vi "sub_simulation_main.vi"(8 "error in":errorcluster) -> (0 "error out":errorcluster)   [LabVIEW 2016]
uses:
  ctl/UI_cmd-ctl.ctl
  ctl/q_data.ctl
  Global.vi
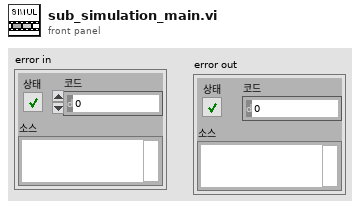
[diagram p1: front panel]
types:
  T1 = typedef "UI_cmd-ctl.ctl" = enum16{"default", "create", "read"}
  T2 = typedef "q_data.ctl" = cluster{"Strain raw wf":waveform(dbl)[], "vacuum raw wf":waveform(dbl), "IR raw 2d":i16[][]}
  T3 = cluster{"simulation file path":path, "simulation speed":u32}
  T4 = typedef "UI_ctl2.ctl" = cluster{"simulation status":refnum<vi>}
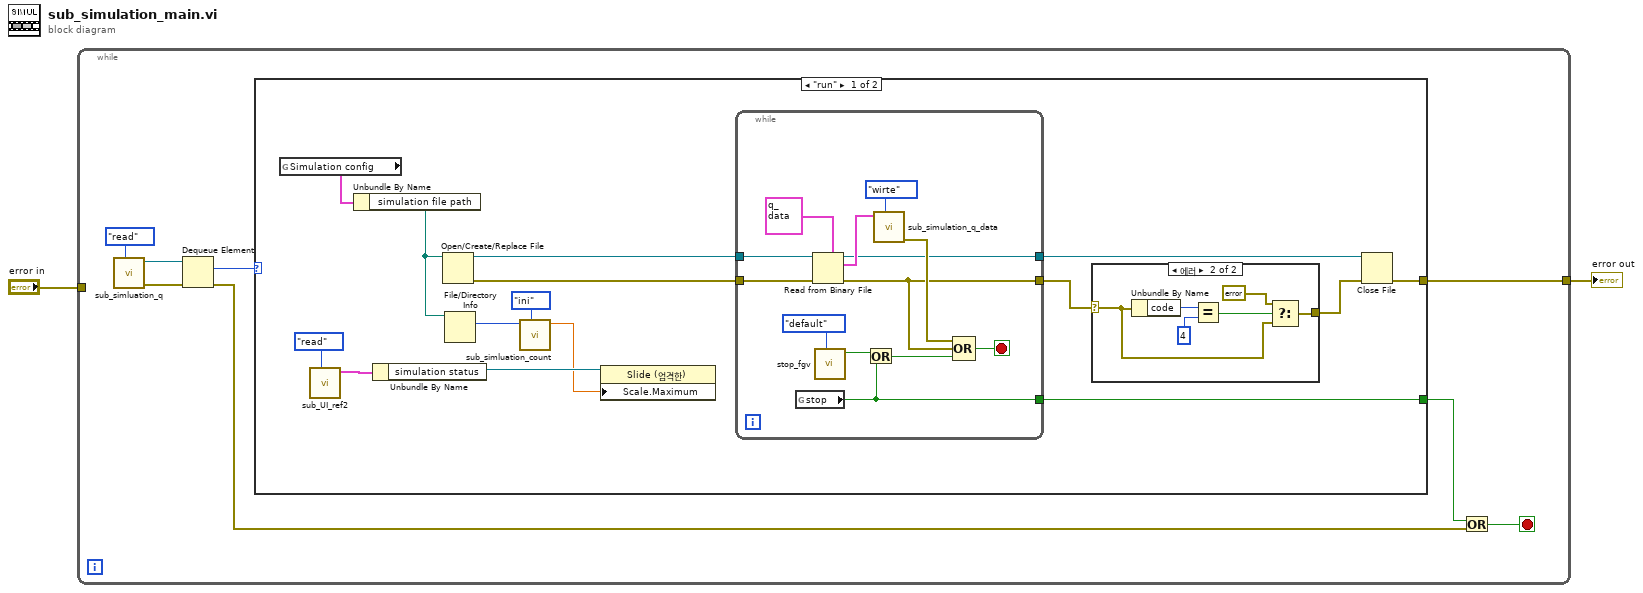
[diagram p0: block diagram]
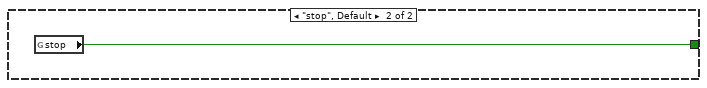
[diagram p3: hidden frame]
diagram:
  n1 = while {
    tunnel: "error in" -> [_]
    tunnel: [w3] -> w1
    stop <- w4 stop-if-true
    n2 = call "sub_simluation_q.vi"("cmd"=enum16{"create", "write", "read", "close"}."read") -> ("error out"=w9:errorcluster, "queue out"=w8:refnum<queue>)  [unwired: 9 in]
    n3 = Dequeue Element(queue=w8, error in (no error)=w9) -> (element=w7:enum16{"run", "stop"}, error out=w5:errorcluster)  [unwired: 1 in, 2 out]
    n4 = case shown="\"run\"" w7 {
      tunnel: [w22 w46] -> w6
      tunnel: [w21 _] -> w3
      frame "run" {
        n5 = global read "Global.vi" "Simulation config"() -> (w18:T3)
        n6 = call "sub_UI_ref2.vi"("cmd"=UI_cmd-ctl."read") -> ("UI ctl2 out"=w15:T4)  [unwired: 10 in]
        n7 = Unbundle By Name(w18) -> ("simulation file path"=w17:path)
        n8 = Unbundle By Name(w15) -> ("simulation status"=w14:refnum<vi>)
        n9 = Open/Create/Replace File(file path (use dialog)=w17) -> (refnum out=w23:refnum<file>, error out=w25:errorcluster)  [unwired: 5 in, 1 out]
        n10 = File/Directory Info(path=w17) -> (size=w13:i64)  [unwired: 1 in, 6 out]
        n11 = call "sub_simluation_count.vi"("cmd"=enum16{"ini", "count"}."ini", "data"=w13) -> ("max"=w11:dbl)  [unwired: 8 in, 1 out]
        n12 = property class="Slide (엄격한)"(reference=w14, "Scale.Maximum"=w11) -> ()  [unwired: 1 in, 2 out]
        n13 = while {
          tunnel: w25 -> [w45]
          tunnel: [w35] -> w20
          tunnel: [w34] -> w24
          tunnel: w23 -> [w36]
          tunnel: [w37] -> w22
          stop <- w39 stop-if-true
          n14 = global read "Global.vi" "stop"() -> (w37:bool)
          n15 = Read from Binary File(5:T2 {"Strain raw wf"=[], "vacuum raw wf"={"t0"=timestamp(0 s since 1904-01-01), "dt"=1.0, "Y"=[]}, "IR raw 2d"=[]} ("Q_data"), 8:w45, 11:w36) -> (0:w35:errorcluster, 2:w42:T2, 3:w34:refnum<file>)  [unwired: 3 in, 1 out]
          n16 = call "stop_fgv.vi"("cmd"=enum16{"default", "ini", "stop"}."default") -> ("stop"=w38:bool)  [unwired: 9 in, 1 out]
          n17 = Or(x=w38, y=w37) -> (x .or. y?=w40:bool)
          n18 = call "sub_simulation_q_data.vi"("cmd"=enum16{"create", "wirte", "read", "close"}."wirte", "log data"=w42) -> ("error out"=w41:errorcluster)  [unwired: 8 in, 1 out]
          n19 = Compound Arithmetic op=OR(w41, w35, w40) -> (w39:bool)
        }
        n20 = case shown="에러" w20 {
          selector: w20 -> [w26 w27]
          tunnel: [w26 w28] -> w19
          frame No Error {
          }
          frame Error {
            n21 = Unbundle By Name(w27) -> ("code"=w32:i32)
            n22 = Equal?(x=w32, y=4) -> (x = y?=w30:bool)
            n23 = Select(t=errorcluster {"status"=FALSE, "code"=0, "source"=""} ("error IO"), s=w30, f=w27) -> (s? t:f=w28:errorcluster)
          }
        }
        n24 = Close File(refnum=w24, error in=w19) -> (error out=w21:errorcluster)  [unwired: 1 out]
      }
      frame "stop", Default {
        n25 = global read "Global.vi" "stop"() -> (w46:bool)
      }
    }
    n26 = Or(x=w6, y=w5) -> (x .or. y?=w4:bool)
  }
  "error out" <- w1
